vi "Switch UI.vi"() -> ()   [LabVIEW 2025, in "Switch.lvlib" / "Switch Instrument.lvclass"]
doc: "Copyright 2017 National Instruments Corporation\n\nLicensed under the Apache License, Version 2.0 (the \"License\"); you may not use this file except in compliance with the License. You may obtain a copy of the License at http://www.apache.org/licenses/LICENSE-2.0\nUnless required by applicable law or agreed to in writing, software distributed under the License is distributed on an \"AS IS\" BASIS, WITHOUT WARRANTIES OR CONDITIONS OF ANY KIND, either express or implied. See the License for the specific language governing permissions and limitations under the License."
uses:
  Switch Instrument.lvclass
  Switch Instrument.lvclass/Switch Instrument.ctl
  C:/Users/Public/Documents/Sandia National Labs/TSS Plugin/Abstract Engine.lvlibp/Plugin/Abstract/Abstract Instrument/Abstract Instrument.lvclass
  C:/Users/Public/Documents/Sandia National Labs/TSS Plugin/CEF.lvlibp/serializable node/CEF_serializable node.lvclass
  C:/Users/Public/Documents/Sandia National Labs/TSS Plugin/CEF.lvlibp/Node/CEF_Node.lvclass
  C:/Working copy/tss/Plugin/Engines/Switch/Switch Instrument/Switch Instrument.lvclass
  Users/Public/Documents/Sandia National Labs/TSS Plugin/CEF.lvlibp/Node/CEF_Node.lvclass
  Switch configuration/Switch configuration.lvclass
  Users/Public/Documents/Sandia National Labs/TSS Plugin/CEF.lvlibp/Node/NodeRef.ctl
  Users/Public/Documents/Sandia National Labs/TSS Plugin/CEF.lvlibp/Node/UserEventRef.ctl
  Users/Public/Documents/Sandia National Labs/TSS Plugin/CEF.lvlibp/Node/mainQref.ctl
  <instrlib>/niSwitch/niSwitch.llb/niSwitch Topologies.ctl
  Switch configuration/Switch Instrument Setting.ctl
  Users/Public/Documents/Sandia National Labs/TSS Plugin/Abstract Engine.lvlibp/Plugin/Abstract/Instrument configuration/Default Instrument.ctl
  Users/Public/Documents/Sandia National Labs/TSS Plugin/Abstract Engine.lvlibp/Plugin/Abstract/Instrument configuration/Instrument configuration.lvclass
panel:
  in  "DMM":cluster{"Default":T1, "Switch Setting":T2}={"Default"={"Type"="None", "Address"="None", "SW Alias"="None", "Description"="* Type = Class", "Enabled"=TRUE}, "Switch Setting"={"topology name"="Configured Topology"}}
  in  "user event":T4
  in  "main queue":T5
  in  "node ref":T6
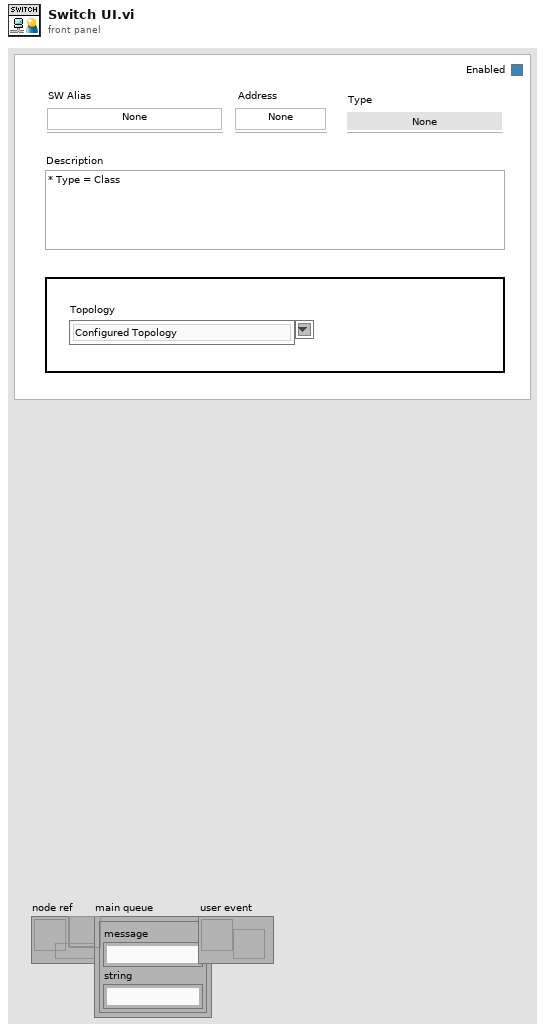
[diagram p1: front panel]
types:
  T1 = typedef "Abstract Engine.lvlibp/Instrument configuration.lvclass/Default Instrument.ctl" = cluster{"Type":string, "Address":string, "SW Alias":string, "Description":string, "Enabled":bool}
  T2 = typedef "Switch.lvlib/Switch configuration.lvclass/Switch Instrument Setting.ctl" = cluster{"topology name":T3}
  T3 = typedef "niSwitch Topologies.ctl" = string
  T4 = typedef "CEF.lvlibp/CEF_Node.lvclass/UserEventRef.ctl" = refnum<user-event>
  T5 = typedef "CEF.lvlibp/CEF_Node.lvclass/mainQref.ctl" = refnum<queue>
  T6 = typedef "CEF.lvlibp/CEF_Node.lvclass/NodeRef.ctl" = refnum<data-value>
  T7 = cluster{"Type":string, "Address":string, "SW Alias":string, "Description":string, "Enabled":bool}
  T8 = cluster{"Instrument Setting":cluster{"Type":string, "Address":string, "SW Alias":string, "Description":string, "Enabled":bool}, "Switch Setting":T2}
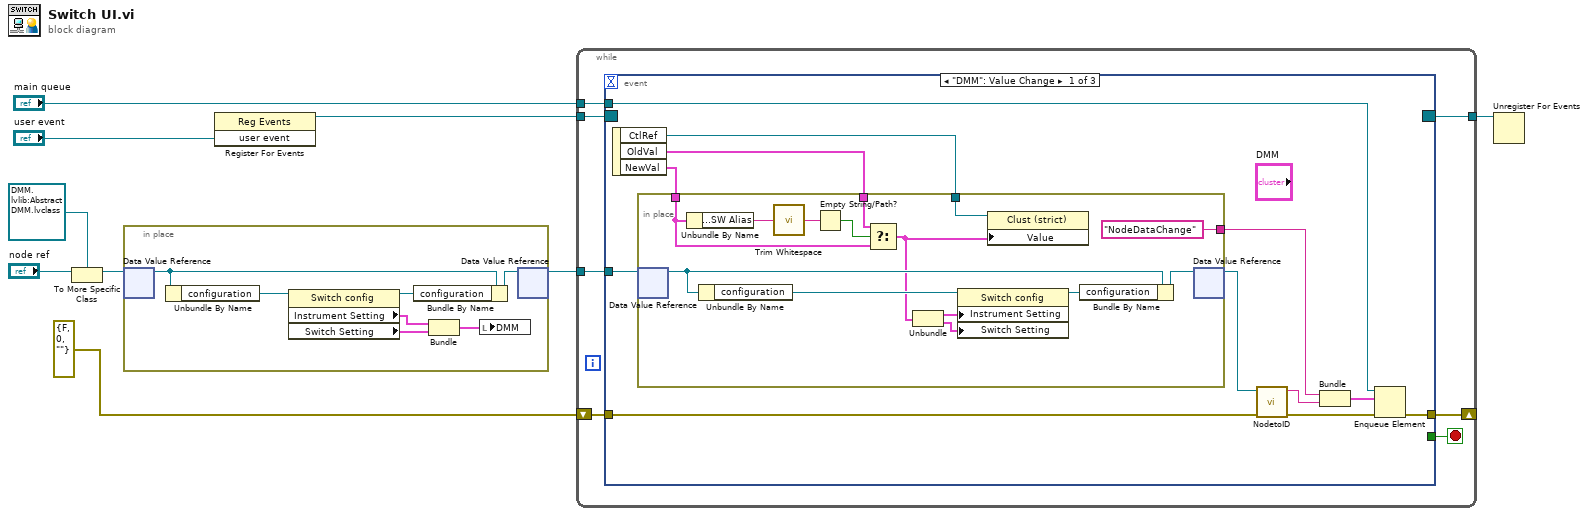
[diagram p0: block diagram]
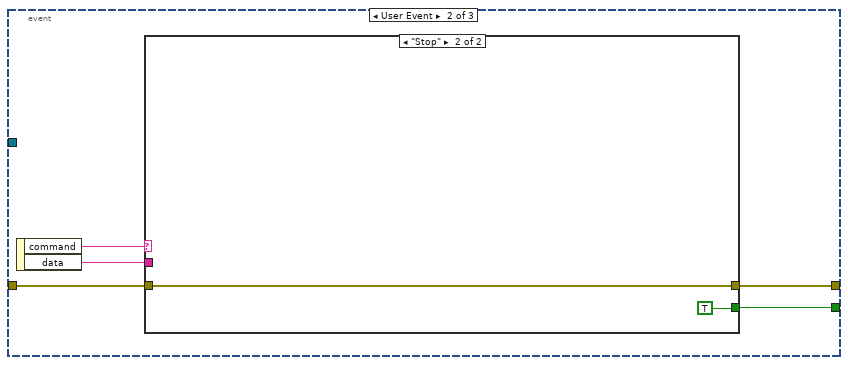
[diagram p2: hidden frame]
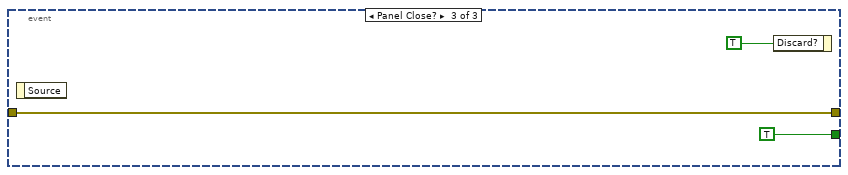
[diagram p4: hidden frame]
diagram:
  n1 = To More Specific Class(target class=refnum<data-value> refnum ("data value reference"), reference="node ref") -> (specific class reference=w6:refnum<data-value>)  [unwired: 1 in, 1 out]
  n2 = in-place {
    # "Initialize the front panel controls when loaded"
    n3 = in-place-dvr #1(w6) -> (w15:refnum<class "Switch Instrument.lvclass">)  [unwired: 1 out]
    n4 = Unbundle By Name(w15) -> ("configuration"=w16:refnum<class "Switch configuration.lvclass">)
    n5 = property class="Switch config"(reference=w16) -> (reference out=w14:refnum<class "Switch configuration.lvclass">, "Instrument Setting"=w12:T7, "Switch Setting"=w11:T2)  [unwired: 1 in, 1 out]
    n6 = Bundle By Name(cluster=w15, "configuration"=w14) -> (w13:refnum<class "Switch Instrument.lvclass">)
    n7 = Bundle("Instrument Setting"=w12, "Switch Setting"=w11) -> (w10:T8)  [unwired: 1 in]
    n8 = local write "DMM"(w10) -> ()
    n9 = in-place-dvr #1(w13) -> (w5:refnum<data-value>)  [unwired: 1 out]
  }
  n10 = register-events("user event") -> (reference out=w9:refnum<event-registration>)  [unwired: 2 in, 1 out]
  n11 = while {
    tunnel: w5 -> [w23]
    tunnel: w9 -> [w22]
    tunnel: [w21] -> w8
    tunnel: "main queue" -> [w17]
    shift-right: [w18] -> _
    shift-left: errorcluster {"status"=FALSE, "code"=0, "source"=""} ("error out") -> [w19]
    stop <- w20 stop-if-true
    n12 = event shown="[0] \"DMM\": Value Change" {
      selector: w22 -> [_ _ _]
      dyn-events: [_ _ _] -> w21
      timeout: _ -> [_ _ _]
      tunnel: w23 -> [w31 _ _]
      tunnel: [_ w54 TRUE] -> w20
      tunnel: [w32 w50 w59] -> w18
      tunnel: w19 -> [w33 w52 w59]
      tunnel: w17 -> [w34 _ _]
      event "DMM": Value Change {
        n13 = event-data() -> ("CtlRef"=w27:refnum<vi>, "OldVal"=w28:cluster{"Default":T1, "Switch Setting":T2}, "NewVal"=w29:cluster{"Default":T1, "Switch Setting":T2})  [unwired: 1 in]
        n14 = in-place {
          in-place-border: w29 -> [w44]
          in-place-border: w28 -> [w42]
          in-place-border: w27 -> [w41]
          in-place-border: ["NodeDataChange" ("Message Name")] -> w26
          n15 = in-place-dvr #2(w31) -> (w49:refnum<class "Switch Instrument.lvclass">)  [unwired: 1 out]
          n16 = Unbundle By Name(w44) -> ("Default.SW Alias"=w45:string)
          n17 = Unbundle By Name(w49) -> ("configuration"=w48:refnum<class "Switch configuration.lvclass">)
          n18 = call <vilib>:"Trim Whitespace.vi"("string"=w45) -> ("trimmed string"=w40:string)  [unwired: 1 in]
          n19 = Empty String/Path?(string/path=w40) -> (empty?=w43:bool)
          n20 = Select(t=w42, s=w43, f=w44) -> (s? t:f=w39:cluster{"Default":T1, "Switch Setting":T2})
          n21 = Unbundle(w39) -> ("Default"=w38:T1, "Switch Setting"=w37:T2)
          n22 = property class="Switch config"(reference=w48, "Instrument Setting"=w38, "Switch Setting"=w37) -> (reference out=w46:refnum<class "Switch configuration.lvclass">)  [unwired: 1 in, 1 out]
          n23 = property class="Clust (strict)"(reference=w41, "Value"=w39) -> ()  [unwired: 1 in, 2 out]
          n24 = Bundle By Name(cluster=w49, "configuration"=w46) -> (w47:refnum<class "Switch Instrument.lvclass">)
          n25 = in-place-dvr #2(w47) -> (w30:refnum<data-value>)  [unwired: 1 out]
        }
        n26 = call "NodetoID.vi"("error in"=w33, "node ref"=w30) -> ("error out"=w35:errorcluster, "ID"=w25:string)  [unwired: 8 in]
        n27 = Bundle("Message Name"=w26, "ID"=w25) -> (w24:cluster{"Message Name":string, "ID":string})  [unwired: 1 in]
        n28 = Enqueue Element(queue=w34, element=w24, error in (no error)=w35) -> (error out=w32:errorcluster)  [unwired: 1 in, 2 out]
      }
      event User Event {
        n29 = event-data() -> ("command"=w51:string, "data"=w53:string)  [unwired: 1 in]
        n30 = case shown="\"Stop\"" w51 {
          tunnel: [_ TRUE] -> w54
          tunnel: w53 -> [_ _]
          tunnel: w52 -> [w55 w56]
          tunnel: [w55 w56] -> w50
          frame Default {
          }
          frame "Stop" {
          }
        }
      }
      event Panel Close? {
        n31 = event-data() -> ()  [unwired: 1 in, 1 out]
        n32 = event-data("Discard?"=TRUE) -> ()  [unwired: 1 in, 1 out]
      }
    }
  }
  n33 = Unregister For Events(event registration refnum=w8) -> ()  [unwired: 1 in, 1 out]
